vi "Build Description String.vi"(8 "error in (no error)":errorcluster, 11 "Mouse Action in":refnum<class "Mouse Action.lvclass">) -> (0 "error out":errorcluster, 2 "Description":string, 3 "Mouse Action out":refnum<class "Mouse Action.lvclass">)   [LabVIEW 2020, in "MacroAssert.lvlib" / "Mouse Action.lvclass"]
doc: "Builds a string to describe what <B>Step</B> does."
uses:
  Mouse Action.lvclass
  Action Step/Action Step.lvclass
  Mouse Action.lvclass/Mouse Action.ctl
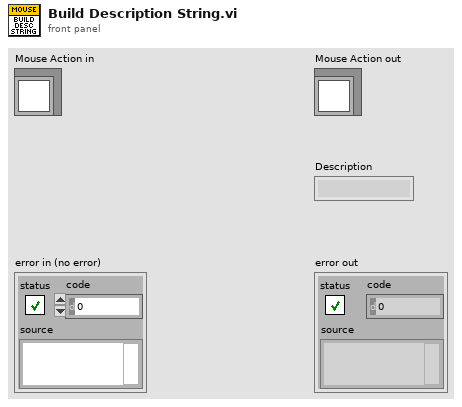
[diagram p1: front panel]
types:
  T1 = typedef "MacroAssert.lvlib/Mouse Action.lvclass/Mouse Action Type.ctl" = enum16{"Click", "Absolute Move", "Absolute Move and Click", "Relative Move", "Relative Move and Click", "Wheel Up", "Wheel Down"}
  T2 = typedef "MacroAssert.lvlib/Mouse Action.lvclass/Button.ctl" = enum16{"Left", "Right", "Middle"}
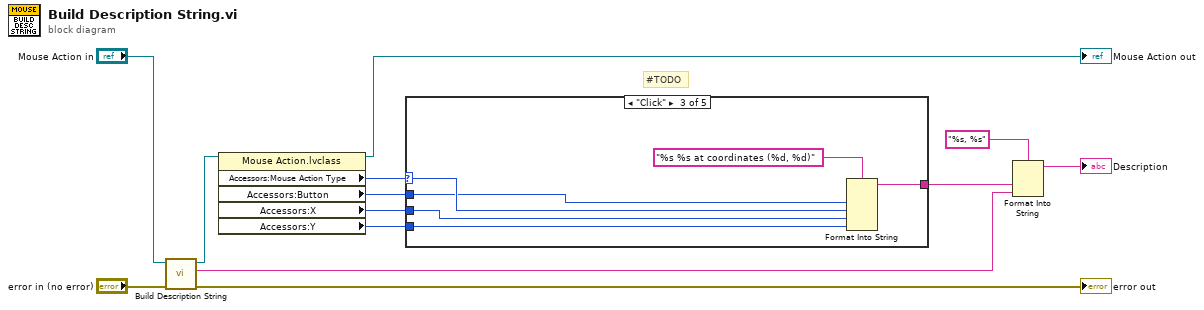
[diagram p0: block diagram]
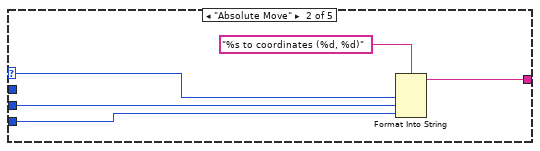
[diagram p3: hidden frame]
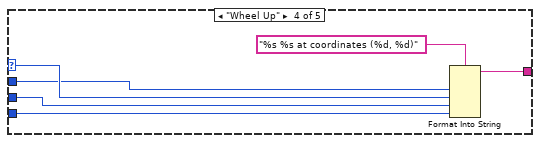
[diagram p4: hidden frame]
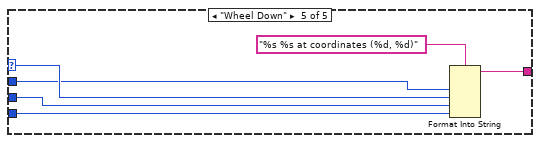
[diagram p5: hidden frame]
diagram:
  # "#TODO"
  n1 = call-parent "Build Description String.vi"("error in (no error)"="error in (no error)", "Action Step in"="Mouse Action in") -> ("error out"=→"error out":errorcluster, "Description"=w2:string, "Action Step out"=w6:refnum<class "Mouse Action.lvclass">)  [unwired: 7 in]
  n2 = property class="Mouse Action.lvclass"(reference=w6) -> (reference out=→"Mouse Action out":refnum<class "Mouse Action.lvclass">, "Accessors:Mouse Action Type"=w10:T1, "Accessors:Button"=w1:T2, "Accessors:X"=w12:i32, "Accessors:Y"=w11:i32)  [unwired: 1 in, 1 out]
  n3 = case shown="\"Click\"" w10 {
    selector: w10 -> [_ w14 w20 w26 w32]
    tunnel: [_ w17 w23 w29 w35] -> w4
    tunnel: w12 -> [_ w16 w22 w28 w34]
    tunnel: w11 -> [_ w15 w21 w27 w33]
    tunnel: w1 -> [_ _ w19 w25 w31]
    frame Default {
    }
    frame "Absolute Move" {
      n4 = Format Into String(format string="%s to coordinates (%d, %d)", w14, w16, w15) -> (resulting string=w17:string)  [unwired: 2 in, 1 out]
    }
    frame "Click" {
      n5 = Format Into String(format string="%s %s at coordinates (%d, %d)", w19, w20, w22, w21) -> (resulting string=w23:string)  [unwired: 2 in, 1 out]
    }
    frame "Wheel Up" {
      n6 = Format Into String(format string="%s %s at coordinates (%d, %d)", w25, w26, w28, w27) -> (resulting string=w29:string)  [unwired: 2 in, 1 out]
    }
    frame "Wheel Down" {
      n7 = Format Into String(format string="%s %s at coordinates (%d, %d)", w31, w32, w34, w33) -> (resulting string=w35:string)  [unwired: 2 in, 1 out]
    }
  }
  n8 = Format Into String(format string="%s, %s", w4, w2) -> (resulting string=→"Description":string)  [unwired: 2 in, 1 out]
